vi "unflatten switch config.vi"(8 "error in (no error)":errorcluster, 10 "Motion Switch Array in":T1[](array[typedef]), 11 "string":string) -> (0 "error out":errorcluster, 3 "Motion Switch Array out":T1[](array[typedef]))   [LabVIEW 2018]
uses:
  02.Type Def's/All Switch Configuration Cluster.ctl
  02.Type Def's/All Motions.ctl
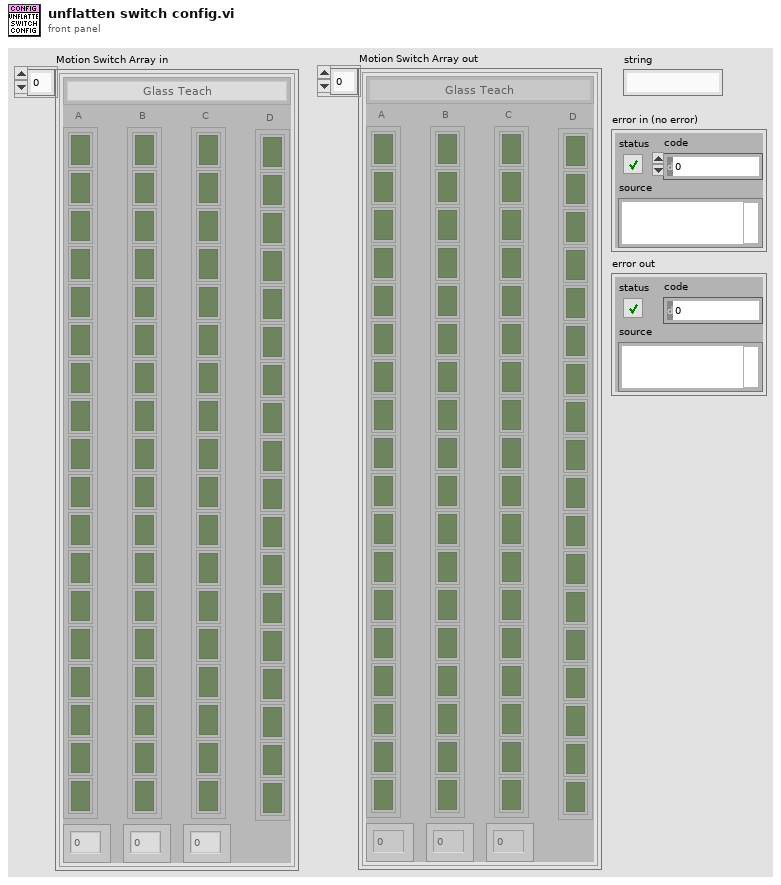
[diagram p1: front panel]
types:
  T1 = typedef "All Switch Configuration Cluster.ctl" = cluster{"All Motions":T2, "A":bool[], "B":bool[], "C":bool[], "D":bool[], "A activation time (ms)":u32, "B activation time (ms)":u32, "C activation time (ms)":u32}
  T2 = typedef "All Motions.ctl" = enum16{"Glass Teach", "Glass Slide Open", "Glass Slide Close", "Glass Vent Open", "Glass Vent Close", "Sunshade Teach", "Sunshade Open", "Sunshade Close", "Idle", "Sunshade Open 2", "Sunshade Close 2", "Glass Slide Open Sunshade Open", "Glass Slide Open Sunshade Close", "Glass Slide Close Sunshade Open", "Glass Slide Close Sunshade Close", "Glass Vent Open Sunshade Open", "Glass Vent Open Sunshade Close", "Glass Vent Close Sunshade Open", "Glass Vent Close Sunshade Close", "Express Glass Slide Open", "Express Glass Slide Close", "Express Glass Vent Open", "Express Glass Vent Close", "Express Sunshade Open", "Express Sunshade Close", "Express Sunshade Open 2", "Express Sunshade Close 2", "Express Glass Slide Open Sunshade Open", "Express Glass Slide Open Sunshade Close", "Express Glass Slide Close Sunshade Open", "Express Glass Slide Close Sunshade Close", "Express Glass Vent Open Sunshade Open", "Express Glass Vent Open Sunshade Close", "Express Glass Vent Close Sunshade Open", "Express Glass Vent Close Sunshade Close", "Goto Position Glass", "Goto Position Sunshade", "Sunshade Teach 2"}
  T3 = cluster{"All Motions":enum16{"Glass Teach", "Glass Slide Open", "Glass Slide Close", "Glass Vent Open", "Glass Vent Close", "Sunshade Teach", "Sunshade Open", "Sunshade Close", "Idle", "Sunshade Open 2", "Sunshade Close 2", "Glass Slide Open Sunshade Open", "Glass Slide Open Sunshade Close", "Glass Slide Close Sunshade Open", "Glass Slide Close Sunshade Close", "Glass Vent Open Sunshade Open", "Glass Vent Open Sunshade Close", "Glass Vent Close Sunshade Open", "Glass Vent Close Sunshade Close", "Express Glass Slide Open", "Express Glass Slide Close", "Express Glass Vent Open", "Express Glass Vent Close", "Express Sunshade Open", "Express Sunshade Close", "Express Sunshade Open 2", "Express Sunshade Close 2", "Express Glass Slide Open Sunshade Open", "Express Glass Slide Open Sunshade Close", "Express Glass Slide Close Sunshade Open", "Express Glass Slide Close Sunshade Close", "Express Glass Vent Open Sunshade Open", "Express Glass Vent Open Sunshade Close", "Express Glass Vent Close Sunshade Open", "Express Glass Vent Close Sunshade Close", "Goto Position Glass", "Goto Position Sunshade"}, "A":bool[], "B":bool[], "C":bool[], "D":bool[]}[]
  T4 = enum16{"Glass Teach", "Glass Slide Open", "Glass Slide Close", "Glass Vent Open", "Glass Vent Close", "Sunshade Teach", "Sunshade Open", "Sunshade Close", "Idle", "Sunshade Open 2", "Sunshade Close 2", "Glass Slide Open Sunshade Open", "Glass Slide Open Sunshade Close", "Glass Slide Close Sunshade Open", "Glass Slide Close Sunshade Close", "Glass Vent Open Sunshade Open", "Glass Vent Open Sunshade Close", "Glass Vent Close Sunshade Open", "Glass Vent Close Sunshade Close", "Express Glass Slide Open", "Express Glass Slide Close", "Express Glass Vent Open", "Express Glass Vent Close", "Express Sunshade Open", "Express Sunshade Close", "Express Sunshade Open 2", "Express Sunshade Close 2", "Express Glass Slide Open Sunshade Open", "Express Glass Slide Open Sunshade Close", "Express Glass Slide Close Sunshade Open", "Express Glass Slide Close Sunshade Close", "Express Glass Vent Open Sunshade Open", "Express Glass Vent Open Sunshade Close", "Express Glass Vent Close Sunshade Open", "Express Glass Vent Close Sunshade Close", "Goto Position Glass", "Goto Position Sunshade"}
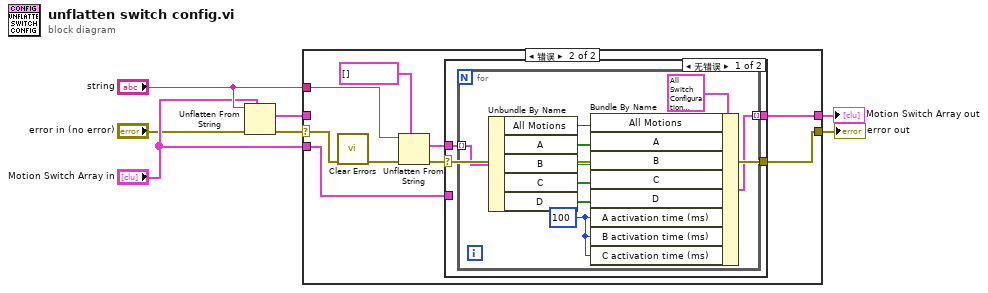
[diagram p0: block diagram]
diagram:
  n1 = Unflatten From String(type="Motion Switch Array in", binary string="string", error in (no error)="error in (no error)") -> (value=w6:T1[], error out=w5:errorcluster)  [unwired: 2 in, 1 out]
  n2 = case shown="错误" w5 {
    selector: w5 -> [w8 w17]
    tunnel: "Motion Switch Array in" -> [_ w12]
    tunnel: w6 -> [w9 _]
    tunnel: [w9 w14] -> w4
    tunnel: "string" -> [_ w10]
    tunnel: [w8 w11] -> w1
    frame No Error {
    }
    frame Error {
      n3 = call <vilib>:"Clear Errors.vi"("error in (no error)"=w17) -> ("error out"=w16:errorcluster)  [unwired: 5 in, 1 out]
      n4 = Unflatten From String(type=T3 [] ("Motion Switch Array"), binary string=w10, error in (no error)=w16) -> (value=w15:T3, error out=w13:errorcluster)  [unwired: 2 in, 1 out]
      n5 = case shown="无错误" w13 {
        selector: w13 -> [w19 w31]
        tunnel: w15 -> [w21 _]
        tunnel: [w20 w32] -> w14
        tunnel: w12 -> [_ w32]
        tunnel: [w19 w31] -> w11
        frame No Error {
          n6 = for {
            tunnel: w21 -> [w30] mode=indexing
            tunnel: [w22] -> w20 mode=indexing
            w23 = u32 100 ("A activation time (ms)")
            n7 = Unbundle By Name(w30) -> ("All Motions"=w28:T4, "A"=w27:bool[], "B"=w26:bool[], "C"=w25:bool[], "D"=w24:bool[])
            n8 = Bundle By Name(cluster=T1 {"All Motions"=enum."Glass Teach", "A"=[], "B"=[], "C"=[], "D"=[], "A activation time (ms)"=0, "B activation time (ms)"=0, "C activation time (ms)"=0} ("All Switch Configuration Cluster"), "All Motions"=w28, "A"=w27, "B"=w26, "C"=w25, "D"=w24, "A activation time (ms)"=w23, "B activation time (ms)"=w23, "C activation time (ms)"=w23) -> (w22:T1)
          }
        }
        frame Error {
        }
      }
    }
  }
  "Motion Switch Array out" <- w4
  "error out" <- w1
